vi "SP_WAITLOOP.vi"(3 "Commands":string[](array[string])) -> (1 "Commands Out":string[](array[string]))   [LabVIEW 2009]
panel:
  # "This LabVIEW item is deprecated.\n\nIt is believed to be unused and will be removed in a future version of SRV."
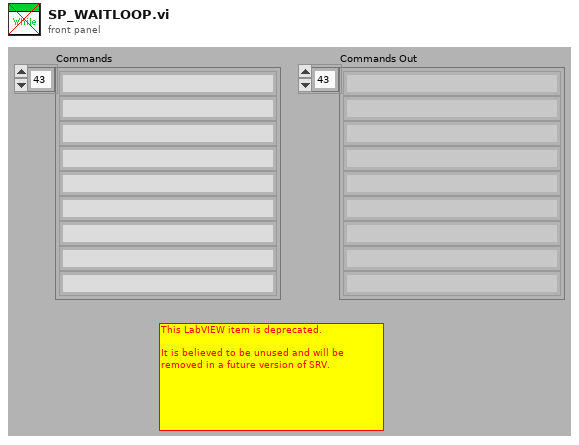
[diagram p1: front panel]
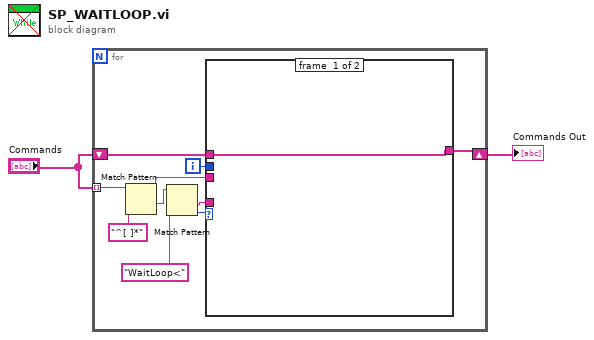
[diagram p0: block diagram]
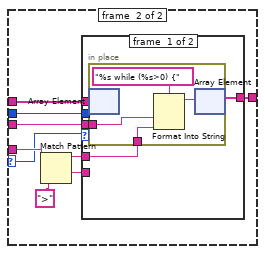
[diagram p2: hidden frame]
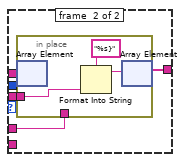
[diagram p3: hidden frame]
diagram:
  n1 = for {
    tunnel: "Commands" -> [w7] mode=indexing
    shift-right: [w8] -> w1
    shift-left: "Commands" -> [w10]
    i -> [w9]
    n2 = Match Pattern(string=w7, regular expression="^[ ]*") -> (match substring=w4:string, after substring=w6:string)  [unwired: 1 in, 2 out]
    n3 = Match Pattern(string=w6, regular expression="WaitLoop<") -> (after substring=w11:string, offset past match=w3:i32)  [unwired: 1 in, 2 out]
    n4 = case shown="Default" w3 {
      selector: w3 -> [_ w14]
      tunnel: w11 -> [_ w19]
      tunnel: w10 -> [w13 w22]
      tunnel: w9 -> [_ w21]
      tunnel: [w13 w20] -> w8
      tunnel: w4 -> [_ w15]
      frame #0 {
      }
      frame #1 {
        n5 = Match Pattern(string=w19, regular expression=">") -> (before substring=w17:string, after substring=w16:string)  [unwired: 1 in, 2 out]
        n6 = case shown="Default" w14 {
          tunnel: w22 -> [w27 w36]
          tunnel: w21 -> [w26 w35]
          tunnel: [w25 w34] -> w20
          tunnel: w17 -> [w24 w33]
          tunnel: w16 -> [_ _]
          tunnel: w15 -> [w23 w32]
          frame #0 {
            n7 = in-place {
              in-place-border: w24 -> [w31]
              in-place-border: w23 -> [w30]
              n8 = in-place-array #1(w27, w26) -> ()  [unwired: 1 out]
              n9 = Format Into String(format string="%s while (%s>0) {", w30, w31) -> (resulting string=w29:string)  [unwired: 2 in, 1 out]
              n10 = in-place-array #1(w29) -> (w25:string[])  [unwired: 1 out]
            }
          }
          frame #1 {
            n11 = in-place {
              in-place-border: w33 -> [_]
              in-place-border: w32 -> [w39]
              n12 = in-place-array #2(w36, w35) -> ()  [unwired: 1 out]
              n13 = Format Into String(format string="%s}", w39) -> (resulting string=w38:string)  [unwired: 2 in, 1 out]
              n14 = in-place-array #2(w38) -> (w34:string[])  [unwired: 1 out]
            }
          }
        }
      }
    }
  }
  "Commands Out" <- w1
